vi "Test Pass.vi"(11 "Test Case In":refnum<class "Fail.lvclass">) -> (0 "error out":errorcluster, 3 "Test Case Out":refnum<class "Fail.lvclass">)   [LabVIEW 2020, in "Fail.lvclass"]
uses:
  Fail.lvclass
  C:/git/astemes-lunit/source/LUnit Test Case.lvclass
  source/LUnit Test Case.lvclass/LUnit Test Case.ctl
  4acd223d-b712-4434-8bc5-6d2ce5207c44.vi
  source/Core/LUnit Test Case/Private/Append Pass Result.vi
  source/Core/LUnit Test Case/Private/Append Fail Result.vi
  4acd223d-b712-4434-8bc5-6d2ce5207c44.vi/9c5d11cd-9439-4240-a1ee-d9baace9c924.vi
  source/Core/LUnit Test Case/Private/Run In UI.vi
  <vilib>/Utility/error.llb/Clear Errors.vi
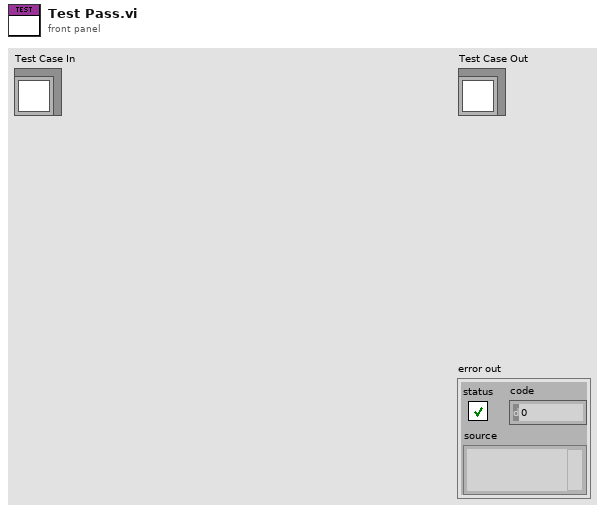
[diagram p1: front panel]
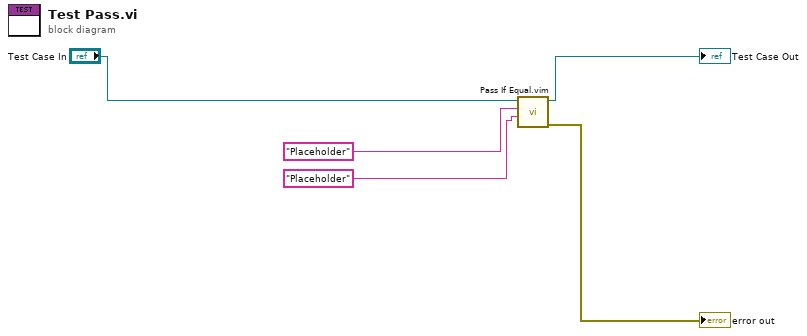
[diagram p0: block diagram]
diagram:
  n1 = call "Pass If Equal.vim"("Actual"="Placeholder", "Expected"="Placeholder", "LUnit Test Case In"="Test Case In") -> ("error out"=→"error out":errorcluster, "LUnit Test Case Out"=→"Test Case Out":refnum<class "Fail.lvclass">)  [unwired: 7 in]
